vi "Change voltages to kg.vi"(11 "Array":dbl[](array[numeric])) -> (1 "Numeric":dbl, 2 "Boolean":bool, 3 "Numeric 2":dbl, 4 "Waveform Chart":dbl[](graph))   [LabVIEW 2016]
uses:
  <vilib>/Analysis/NI_AALBase.lvlib
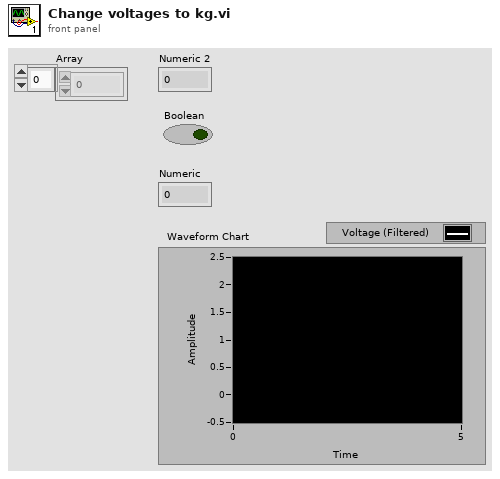
[diagram p1: front panel]
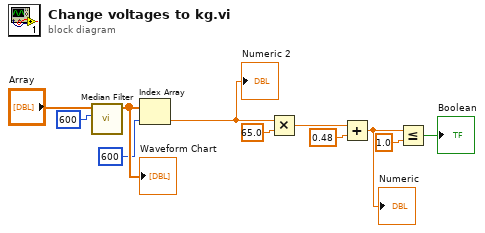
[diagram p0: block diagram]
diagram:
  n1 = call <vilib>:"Median Filter.vi"("left rank"=600, "X"="Array") -> ("Filtered X"=w7:dbl[])  [unwired: 8 in, 1 out]
  "Waveform Chart" <- w7
  n2 = Index Array "Index Array"(array=w7, index=600) -> (element=w9:dbl)
  "Numeric 2" <- w9
  n3 = Multiply(x=w9, y=65.0) -> (x*y=w2:dbl)
  n4 = Add(x=w2, y=0.48) -> (x+y=w11:dbl)
  "Numeric" <- w11
  n5 = Less Or Equal?(x=w11, y=1.0) -> (x <= y?=→"Boolean":bool)
